vi "Get Log File Use Time for X-Axis for Continuous Acquisitions.vi"(8 "error in":errorcluster, 11 "log file in":T1 format="%.0x") -> (0 "error out":errorcluster, 2 "use time for x-axis for continuous acquisitions":bool, 3 "log file out":T1 format="%.0x")   [LabVIEW 2027, in "Embedded Data Logger Scripting.lvlib"]
uses:
  Embedded Data Logger Scripting.lvlib
  <vilib>/NI VeriStand/Custom Device API/Custom Device Item Ref.ctl
  Shared/Constants.vi
  <vilib>/NI VeriStand/Custom Device API/Get Item Property (Boolean).vi
  Shared/Embedded Data Logger Shared.lvlib
  <vilib>/NI VeriStand/Custom Device API/Custom Device API.lvlib
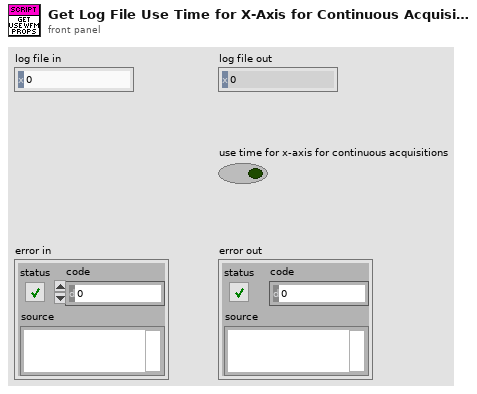
[diagram p1: front panel]
types:
  T1 = typedef "Custom Device API.lvlib/Custom Device Item Ref.ctl" = u64
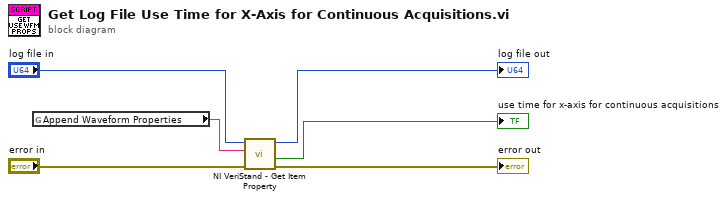
[diagram p0: block diagram]
diagram:
  n1 = global read "Constants.vi" "Append Waveform Properties"() -> (w6:string)
  n2 = call-poly <vilib>:"NI VeriStand - Get Item Property.vi"("error in (no error)"="error in", "Property Name"=w6, "Item Ref in"="log file in") -> ("error out"=→"error out":errorcluster, "Value"=→"use time for x-axis for continuous acquisitions":bool, "Item Ref out"=→"log file out":T1)  [unwired: 5 in, 1 out]
